vi "Lock DB.vi"(8 "error in (no error)":errorcluster, 9 "timeout in ms (-1)":i32, 11 "SQLite in":refnum<class "SQLite.lvclass">) -> (0 "error out":errorcluster, 1 "SQLite DB":refnum<class "Connection.lvclass">, 3 "SQLite out":refnum<class "SQLite.lvclass">, 4 "Timed Out?":bool)   [LabVIEW 2020, in "Summer of LabVIEW.lvlib" / "SQLite.lvclass"]
uses:
  SQLite.lvclass
  SQLite.lvclass/SQLite.ctl
  <vilib>/drjdpowell/SQLite Library/SQL Connection/Connection.lvclass
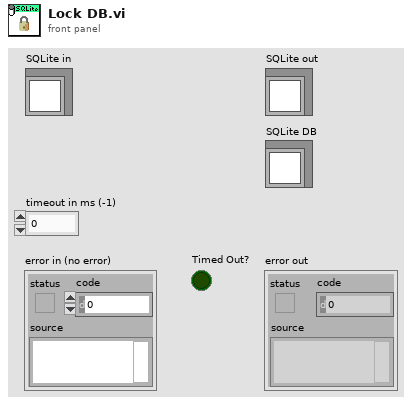
[diagram p1: front panel]
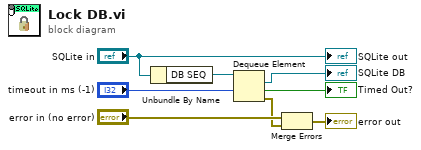
[diagram p0: block diagram]
diagram:
  n1 = Unbundle By Name("SQLite in") -> ("DB SEQ"=w6:refnum<queue>)
  n2 = Dequeue Element(queue=w6, timeout in ms (-1)="timeout in ms (-1)") -> (element=→"SQLite DB":refnum<class "Connection.lvclass">, timed out?=→"Timed Out?":bool, error out=w3:errorcluster)  [unwired: 1 in, 1 out]
  n3 = Merge Errors("error in (no error)", w3) -> (→"error out":errorcluster)
  "SQLite out" <- "SQLite in"
